vi "Lakeshore 336.vi"() -> (0 "Sensor Data":dbl format="%.4f")   [LabVIEW 2023]
uses:
  <instrlib>/Lake Shore 336/Public/Data/Sensor Data (Single Reading).vi
  Global temperature.vi
  <instrlib>/Lake Shore 336/Lake Shore 336.lvlib
panel:
  out "%":dbl
  in  "Ramp":dbl
  in  "Ramp":bool
  out "Actual setpoint":dbl format="%.4f"
  in  "Heater":u16(ring) items=["Off", "Low", "Medium", "High"]
  in  "set":bool
  in  "Setpoint":dbl
  in  "stop":bool
  out "Temperature Chart":dbl(graph)
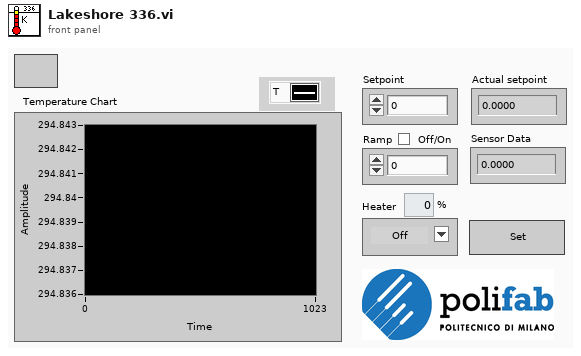
[diagram p1: front panel]
types:
  T1 = cluster{"Baud Rate":u32, "Parity":u16, "Data Bits":u16, "Stop Bits":u16, "Flow Control":u16}
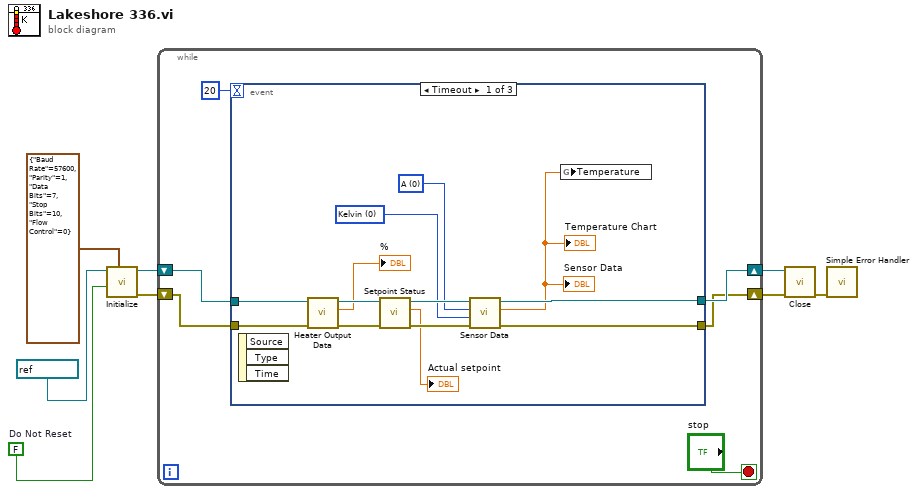
[diagram p0: block diagram]
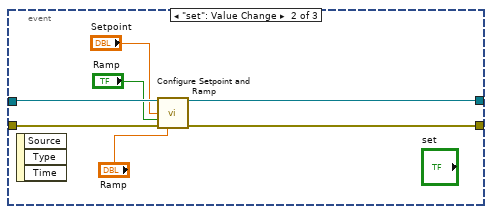
[diagram p2: hidden frame]
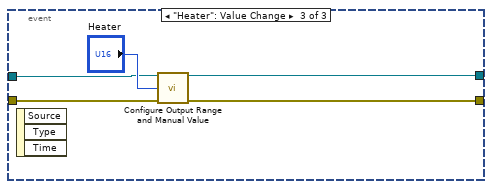
[diagram p3: hidden frame]
diagram:
  w7 = FALSE  # Do Not Reset
  n1 = call <instrlib>:"Initialize.vi"("Serial Configuration"=T1 {"Baud Rate"=57600, "Parity"=1, "Data Bits"=7, "Stop Bits"=10, "Flow Control"=0}, "Reset (True)"=w7, "VISA resource name"=refnum<visa-resource-name> "COM3") -> ("error out"=w2:errorcluster, "VISA resource name out"=w3:refnum<visa-resource-name>)  [unwired: 7 in]
  n2 = while {
    shift-right: [w14] -> w5
    shift-left: w3 -> [w12]
    shift-right: [w13] -> w4
    shift-left: w2 -> [w11]
    stop <- "stop" stop-if-true
    n3 = event shown="[0] Timeout" {
      selector: _ -> [_ _ _]
      dyn-events: _ -> [_ _ _]
      timeout: u32 20 ("milliseconds to wait") -> [_ _ _]
      tunnel: [w27 w30 w37] -> w14
      tunnel: [w26 w32 w36] -> w13
      tunnel: w12 -> [w22 w34 w38]
      tunnel: w11 -> [w19 w33 w35]
      event Timeout {
        w17 = u16 0 items=["Kelvin", "Celsius", "Sensor Units"] ("Data Source (0:Kelvin)")
        w16 = u16 0 items=["A", "B", "C", "D"] ("Input (0:A)")
        n4 = event-data() -> ()  [unwired: 1 in, 3 out]
        n5 = call <instrlib>:"Heater Output Data.vi"("error in (no error)"=w19, "VISA resource name"=w22) -> ("error out"=w20:errorcluster, "Output Value"=→"%":dbl, "VISA resource name out"=w21:refnum<visa-resource-name>)  [unwired: 7 in]
        n6 = call <instrlib>:"Setpoint Status.vi"("error in (no error)"=w20, "VISA resource name"=w21) -> ("error out"=w24:errorcluster, "Setpoint"=→"Actual setpoint":dbl, "VISA resource name out"=w25:refnum<visa-resource-name>)  [unwired: 7 in]
        n7 = call-poly <instrlib>:"Sensor Data.vi"("error in (no error)"=w24, "Data Source (0:Kelvin)"=w17, "Input (0:A)"=w16, "VISA resource name"=w25) -> ("error out"=w26:errorcluster, "Sensor Data"=w15:dbl, "VISA resource name out"=w27:refnum<visa-resource-name>)  [unwired: 5 in]
        "Temperature Chart" <- w15
        "Sensor Data" <- w15
        n8 = global write "Global temperature.vi" "Temperature"(w15) -> ()
      }
      event "set": Value Change {
        n9 = event-data() -> ()  [unwired: 1 in, 3 out]
        n10 = call <instrlib>:"Configure Setpoint and Ramp.vi"("VISA resource name"=w34, "Setpoint (0.00000)"="Setpoint", "Setpoint Ramping \nEnable (F: Off)"="Ramp", "error in (no error)"=w33, "Ramp Rate (0.0)"="Ramp") -> ("VISA resource name out"=w30:refnum<visa-resource-name>, "error out"=w32:errorcluster)  [unwired: 9 in]
      }
      event "Heater": Value Change {
        n11 = event-data() -> ()  [unwired: 1 in, 3 out]
        n12 = call <instrlib>:"Configure Output Range and Manual Value.vi"("VISA resource name"=w38, "Range (0:Off)"="Heater", "error in (no error)"=w35) -> ("VISA resource name out"=w37:refnum<visa-resource-name>, "error out"=w36:errorcluster)  [unwired: 11 in]
      }
    }
  }
  n13 = call <instrlib>:"Close.vi"("error in (no error)"=w4, "VISA resource name"=w5) -> ("error out"=w8:errorcluster)  [unwired: 9 in]
  n14 = call <vilib>:"Simple Error Handler.vi"("error in (no error)"=w8) -> ()  [unwired: 4 in, 5 out]
